vi "Subvi AO mod.vi"(2 "AO channel":refnum<k21>="Connector1/AO0", 10 "Memory label":refnum<k21>="AO0 buffer") -> ()   [LabVIEW 2017]
uses:
  <vilib>/rvi/Emulation/niFpgaGetClockAttributes.vi
  <vilib>/rvi/Emulation/niFpgaSctlEmulationGetInTimedLoop.vi
  <vilib>/rvi/Emulation/niFpgaEmulationReportErrorSimple.vi
  GV buffer-in ready.vi
  Detector/GV line clock start.vi
  <vilib>/rvi/Emulation/niFpgaCriticalErrorInLSC.vi
  <vilib>/rvi/DataTransferAndStorage/Container/Common/niFpgaContainerExecOnDevCompGetState.vi
  <vilib>/rvi/Emulation/niFpgaEmulationIsFPGAContextNoSignature.vi
  <vilib>/rvi/DataTransferAndStorage/Container/Common/niFpgaContainerGetUniqueNameForEmu.vi
  <vilib>/rvi/Emulation/niFpgaProcessEmulError.vi
  <vilib>/rvi/errors/nirviReportUnexpectedCaseInternalError (U32).vi
  <vilib>/rvi/Memory/Memory_Emulation/niFpgaMemoryEmulationCacheClearOnFirstRun.vi
  <vilib>/rvi/Memory/Memory_Emulation/nirvimemoryEmulationManagerCache_MakeExclusive.vi
  <vilib>/rvi/Memory/Memory_Emulation/niFpgaMemoryEmulationValidateCache.vi
  <vilib>/rvi/Memory/Memory_Emulation/nirvimemoryEmulationManagerCache_InsertValue.vi
  <vilib>/Utility/error.llb/Clear Errors.vi
  <vilib>/rvi/Memory/Memory_Emulation/nirvimemoryEmulationManagerCache_ReleaseExclusive.vi
  <vilib>/rvi/Memory/Memory_Emulation/nirvimemoryEmulationManagerCache_GetValue.vi
  <vilib>/rvi/Memory/Memory_Emulation/nirvimemoryEmulationManagerCache_SetValue.vi
  <vilib>/rvi/Emulation/niFpgaSctlEmulationResourceMgr.vi
  <vilib>/rvi/eio/common/nirviEmuTemplateMethod_errors.vi
  <vilib>/rvi/DataTransferAndStorage/Container/XNode/niFpgaContainer.xnode
  <vilib>/rvi/Memory/Memory_Emulation/niFpgaMemoryEmulationRefIn.vi
  <vilib>/eio/EIONode/EIONode.xnode
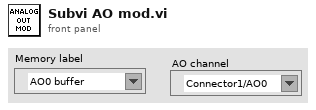
[diagram p1: front panel]
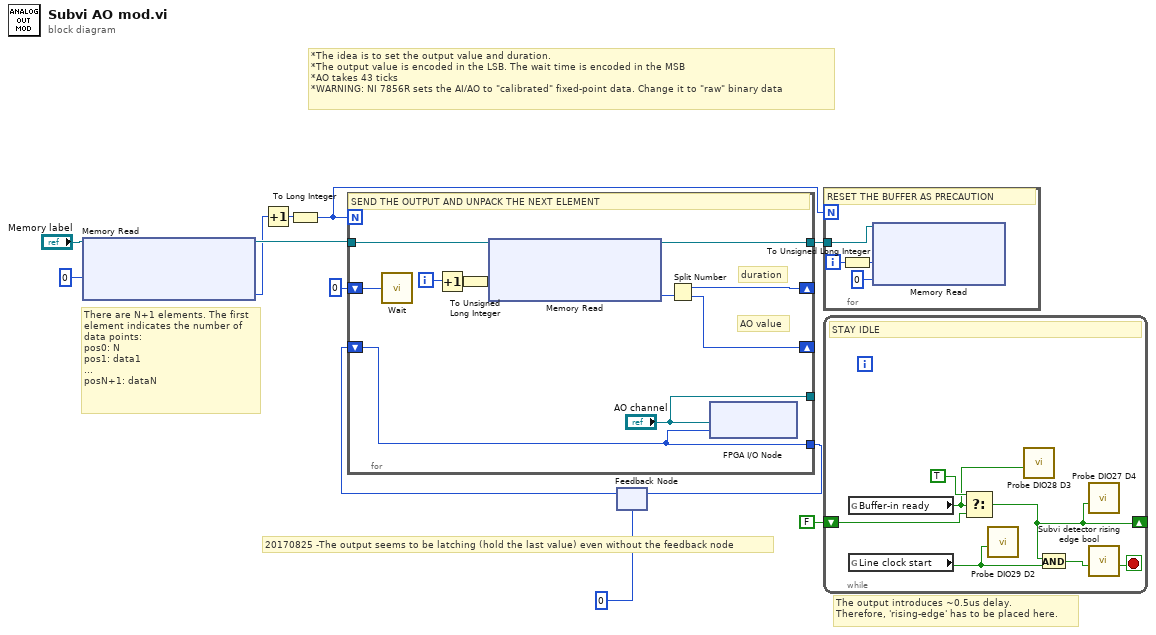
[diagram p0: block diagram]
diagram:
  # "The output introduces ~0.5us delay.\nTherefore, 'rising-edge' has to be placed here."
  # "20170825 -The output seems to be latching (hold the last value) even without the feedback node"
  # "There are N+1 elements. The first\nelement indicates the number of\ndata points:\npos0: N\npos1: data1\n...\nposN+1: dataN"
  # "*The idea is to set the output value and duration.\n*The output value is encoded in the LSB. The wait time is encoded in the MSB\n*AO takes 43 ticks\n*WARNING: NI 7856R sets the AI/AO to \"calibrated\" fixed-point data. Change it to \"raw\" binary data"
  n1 = xnode ("Memory Read")("Address"=u32 0, "Memory In"="Memory label") -> ("Data"=w7:u32, "Memory Out"=w9:refnum<k21>)
  n2 = Increment(x=w7) -> (x+1=w6:u32)
  n3 = To Long Integer(number=w6) -> (32bit integer=w5:i32)
  n4 = feedback #1(u16 0) -> (w4:u16)
  n5 = for {
    N: w5 -> [_]
    shift-right: [w22] -> _
    shift-left: u16 0 -> [w23]
    shift-right: [w20] -> _
    shift-left: w4 -> [w13]
    tunnel: ["AO channel"] -> _
    tunnel: [w19] -> w8
    tunnel: w9 -> [w17]
    tunnel: [w13] -> w2
    i -> [w16]
    # "duration"
    # "AO value"
    # "SEND THE OUTPUT AND UNPACK THE NEXT ELEMENT"
    n6 = call "Wait"("Count(Ticks)"=w23) -> ()  [unwired: 1 out]
    n7 = Increment(x=w16) -> (x+1=w15:i32)
    n8 = To Unsigned Long Integer(number=w15) -> (unsigned 32bit integer=w14:u32)
    n9 = xnode ("Memory Read")("Memory In"=w17, "Address"=w14) -> ("Memory Out"=w19:refnum<k21>, "Data"=w21:u32)
    n10 = Split Number(x=w21) -> (hi(x)=w22:u16, lo(x)=w20:u16)
    n11 = xnode "FPGA I/O Node"("I/O Item"=w13, "FPGA I/O In"="AO channel") -> ()  [unwired: 1 out]
  }
  n12 = feedback-in #1(w2) -> ()
  n13 = for {
    N: w5 -> [_]
    tunnel: w8 -> [w27]
    i -> [w25]
    # "RESET THE BUFFER AS PRECAUTION"
    n14 = To Unsigned Long Integer(number=w25) -> (unsigned 32bit integer=w24:u32)
    n15 = xnode ("Memory Read")("Address"=w24, "Data"=u32 0, "Memory In"=w27) -> ()  [unwired: 1 out]
  }
  n16 = while {
    shift-right: [w28] -> _
    shift-left: FALSE -> [w32]
    stop <- w34 stop-if-true
    # "STAY IDLE"
    n17 = global read "GV buffer-in ready.vi" "Buffer-in ready"() -> (w29:bool)
    n18 = global read "GV line clock start.vi" "Line clock start"() -> (w30:bool)
    n19 = Select(t=TRUE, s=w29, f=w32) -> (s? t:f=w28:bool)
    n20 = call "Probe DIO29 D2.vi"("D2"=w30) -> ()  [unwired: 11 in]
    n21 = call "Probe DIO28 D3.vi"("D3"=w29) -> ()  [unwired: 11 in]
    n22 = And(x=w28, y=w30) -> (x .and. y?=w31:bool)
    n23 = call "Probe DIO27 D4.vi"("D4"=w28) -> ()  [unwired: 11 in]
    n24 = call "Subvi detector rising edge bool.vi"("Input"=w31) -> ("Output"=w34:bool)  [unwired: 10 in]
  }
